vi "PLC.WritePackage.vi"(6 "max package size  (0: full)":i32, 8 "error in (no error)":errorcluster, 9 "data":u8[](array[numeric]), 10 "addr":i32, 11 "Ref in":u64) -> (0 "error out":errorcluster, 3 "Ref out":u64)   [LabVIEW 2016]
doc: "Write data block from PC to PLC\n\nWabco 2017 All right reserved\nAuthor: maciej.szupienko@wabco-auto.com"
panel:
  out "idx":i32
  out "package":u8[](array[numeric])
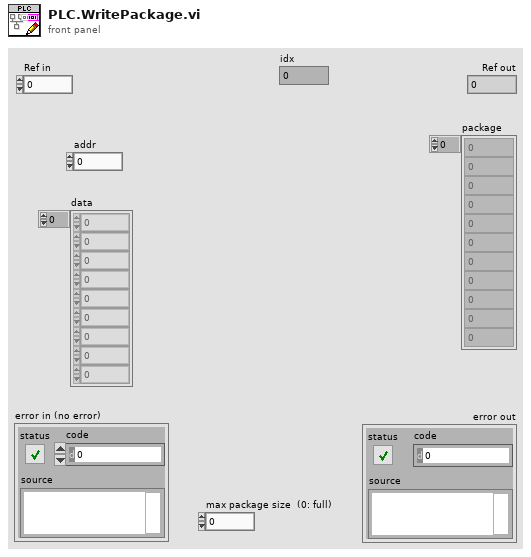
[diagram p1: front panel]
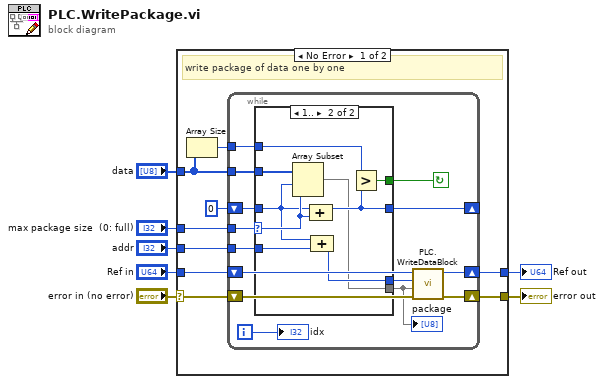
[diagram p0: block diagram]
diagram:
  n1 = case shown="No Error" "error in (no error)" {
    selector: "error in (no error)" -> [w15 w44]
    tunnel: "Ref in" -> [w14 w43]
    tunnel: [w16 w44] -> w6
    tunnel: [w13 w43] -> w5
    tunnel: "data" -> [w10 _]
    tunnel: "addr" -> [w12 _]
    tunnel: "max package size  (0: full)" -> [w11 _]
    frame No Error {
      # "write package of data one by one"
      n2 = Array Size(array=w10) -> (size(s)=w9:i32)
      n3 = while {
        shift-right: [w30] -> w16
        shift-left: w15 -> [w29]
        shift-right: [w27] -> w13
        shift-left: w14 -> [w28]
        tunnel: w10 -> [w26]
        tunnel: w11 -> [w18]
        shift-right: [w24] -> _
        shift-left: 0 -> [w21]
        tunnel: w9 -> [w25]
        tunnel: w12 -> [w22]
        i -> [w19]
        stop <- w23 continue-if-true
        n4 = case shown="1.." w18 {
          selector: w18 -> [_ w36]
          tunnel: w26 -> [w32 w42]
          tunnel: [w32 w35] -> w17
          tunnel: w25 -> [_ w41]
          tunnel: [w33 w40] -> w24
          tunnel: [_ w39] -> w23
          tunnel: w22 -> [w31 w38]
          tunnel: w21 -> [w33 w34]
          tunnel: [w31 w37] -> w20
          frame Default {
          }
          frame 1.. {
            n5 = Array Subset(array=w42, index=w34, length=w36) -> (w35:u8[])
            n6 = Compound Arithmetic op=ADD(w34, w36) -> (w40:i32)
            n7 = Compound Arithmetic op=ADD(w34, w38) -> (w37:i32)
            n8 = Greater?(x=w41, y=w40) -> (0:w39:bool)
          }
        }
        "package" <- w17
        n9 = call "PLC.WriteDataBlock.vi"("error in (no error)"=w29, "data in"=w17, "Block"=w20, "Ref"=w28) -> ("error out"=w30:errorcluster, "ref out"=w27:u64)  [unwired: 6 in]
        "idx" <- w19
      }
    }
    frame Error {
    }
  }
  "error out" <- w6
  "Ref out" <- w5
